vi "SAOMM-SendSET.vi"(0 "PRAMMS-COMM IN":refnum<visa-resource-name>="Hp\u0000\u0002", 1 "Active Refnum":refnum<vi>, 2 "PrAMS-ACK":refnum<vi>, 7 "Signature":u32=1886544237, 11 "Error IN":errorcluster, 12 "MessageType":cluster{string[], u32[]}={["emtError", "emtAreYouThere", "emtAcknowledgment", "emtGetClientType", "emtClientType", "emtGetImageExposureTime", "emtSetImageExposureTime", "emtImageExposureTime", "emtGetOptimalExposureTime", "emtSetOptimalExposureTime", "emtOptimalExposureTime", "emtGetImageEMGain", "emtSetImageEMGain", "emtImageEMGain", "emtGetFPGACtrl", "emtSetFPGACtrl", "emtFPGACtrl", "emtGetImageWidth", "emtSetImageWidth", "emtImageWidth", "emtGetImageHeight", "emtSetImageHeight", "emtImageHeight", "emtGetImageBinning", "emtSetImageBinning", "emtImageBinning", "emtGetImageDisplayFrameRate", "emtSetImageDisplayFrameRate", "emtImageDisplayFrameRate", "emtGetROIWidth", "emtSetROIWidth", "emtROIWidth", "emtGetROIHeight", "emtSetROIHeight", "emtROIHeight", "emtGetROIXOffset", "emtSetROIXOffset", "emtROIXOffset", "emtGetROIYOffset", "emtSetROIYOffset", "emtROIYOffset", "emtStartAcquisition", "mtStopAcquisition", "emtAcquisitionStarted", "emtAcquisitionStopped", "emtGetFalconImage", "emtFalconImage"], [1, 2, 3, 4, 5, 1001, 1101, 1201, 1002, 1102, 1202, 1003, 1103, 1203, 1004, 1104, 1204, 1005, 1105, 1205, 1006, 1106, 1206, 1007, 1107, 1207, 1008, 1108, 1208, 1009, 1109, 1209, 1010, 1110, 1210, 1011, 1111, 1211, 1012, 1112, 1212, 1130, 1131, 1150, 1151, 1070, 1270]}, 13 "Active SET":string="emtSetImageBinning", 14 "Value (little endianed byte array)":u8[](array[numeric])=[2, 0]) -> (4 "PRAMMS-COMM OUT":refnum<visa-resource-name>, 8 "Error":bool, 10 "WaitACKTime":u32=28, 15 "Error OUT":errorcluster)   [LabVIEW 2019]
panel:
  out "CloseTime":u32=5
  out "WriteTime":u32
  out "SortTime":u32
  out "Wait4Flag":u32=27
  out "TotalExec":u32=60
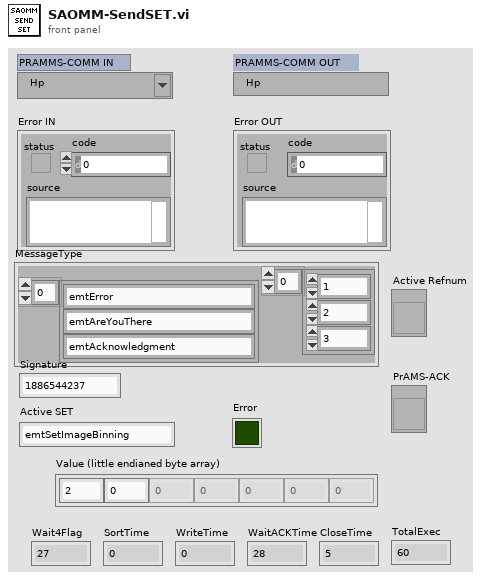
[diagram p1: front panel]
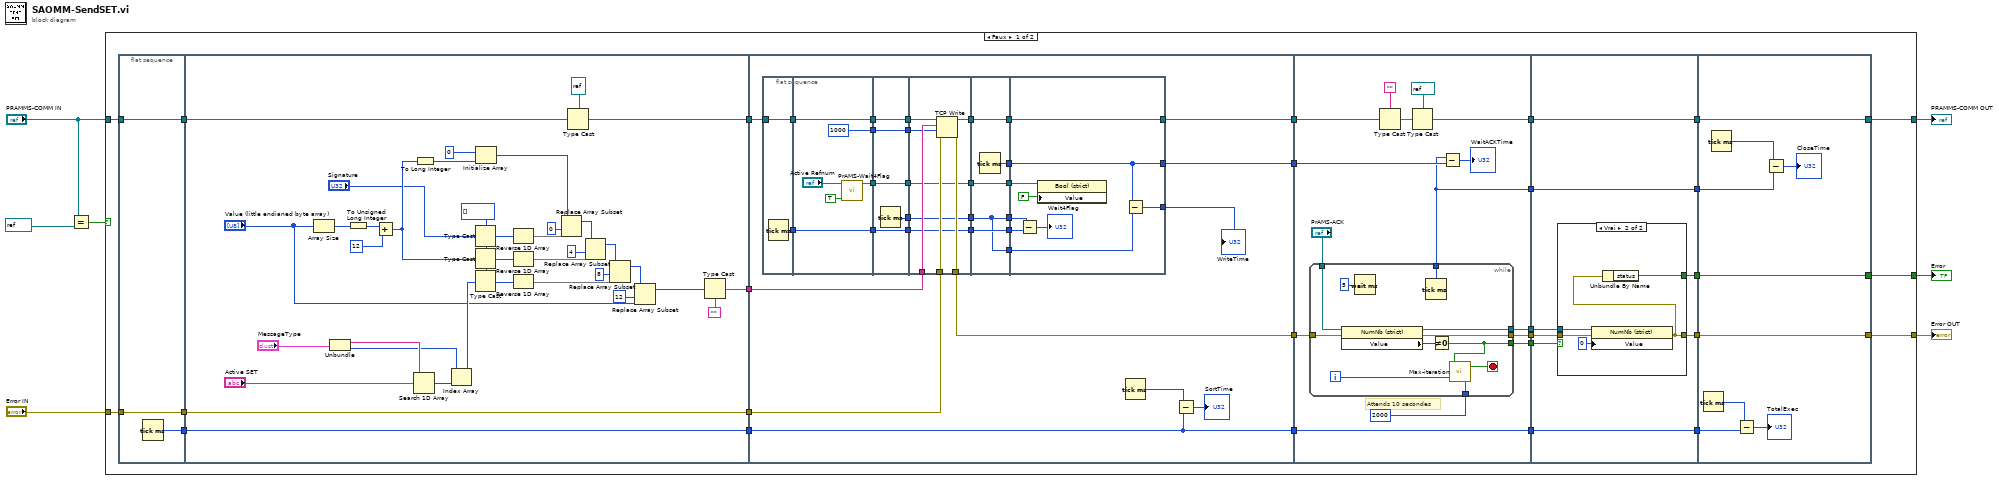
[diagram p0: block diagram]
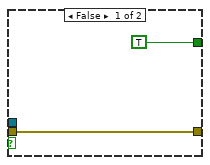
[diagram p2: hidden frame]
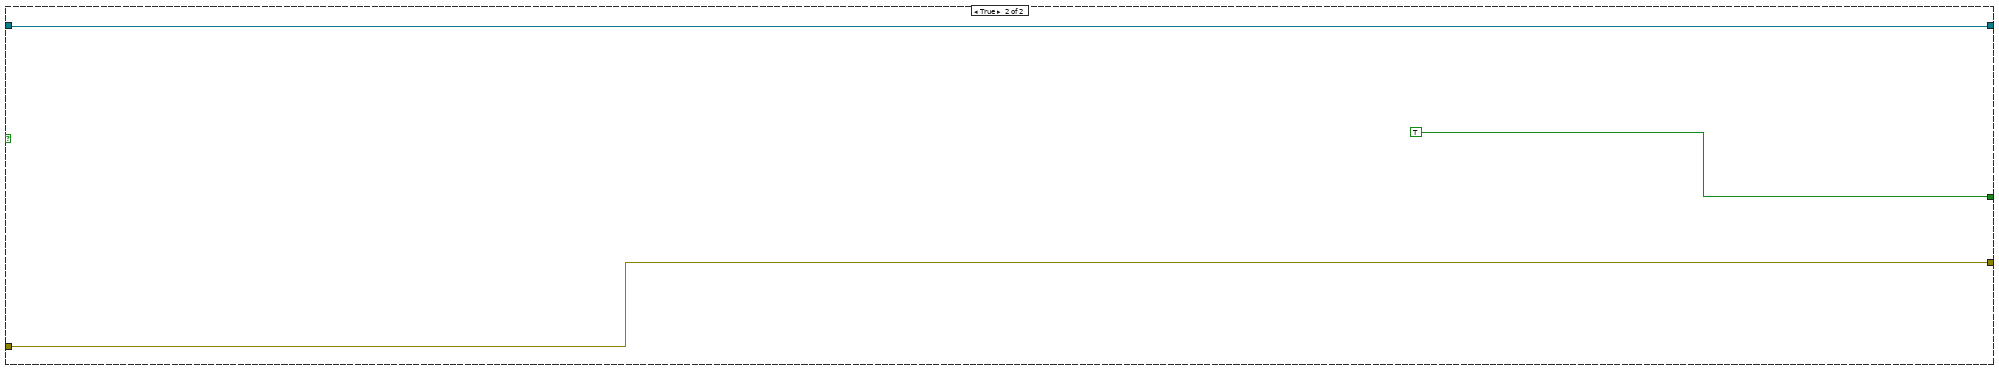
[diagram p3: hidden frame]
diagram:
  n1 = Equal?(x="PRAMMS-COMM IN", y=refnum<visa-resource-name> "-1") -> (x = y?=w4:bool)
  n2 = case shown="Faux" w4 {
    tunnel: "Error IN" -> [w30 w193]
    tunnel: "PRAMMS-COMM IN" -> [w29 w194]
    tunnel: [w28 w193] -> w6
    tunnel: [w14 w194] -> w5
    tunnel: [w27 TRUE] -> w1
    frame False {
      n3 = flat-sequence {
        tunnel: w29 -> [w36]
        tunnel: w30 -> [w37]
        tunnel: [w37] -> w26
        tunnel: [w36] -> w25
        tunnel: [w35] -> w19
        tunnel: w26 -> [w41]
        tunnel: w25 -> [w45]
        tunnel: [w44] -> w16
        tunnel: w19 -> [w44]
        tunnel: [w43] -> w12
        tunnel: [w42] -> w11
        tunnel: [w41] -> w10
        tunnel: [w99] -> w18
        tunnel: [w98] -> w17
        tunnel: w16 -> [w96]
        tunnel: [w96] -> w15
        tunnel: [w103] -> w13
        tunnel: w12 -> [w102]
        tunnel: w11 -> [w101]
        tunnel: w10 -> [w100]
        tunnel: [w156] -> w34
        tunnel: [w155] -> w33
        tunnel: w18 -> [w154]
        tunnel: [w153] -> w32
        tunnel: [w146] -> w31
        tunnel: w17 -> [w151]
        tunnel: [w150] -> w20
        tunnel: w15 -> [w150]
        tunnel: w13 -> [w145]
        tunnel: [w144] -> w8
        tunnel: w34 -> [w174]
        tunnel: w33 -> [w175]
        tunnel: w32 -> [w173]
        tunnel: w31 -> [w171]
        tunnel: [w172] -> w24
        tunnel: [w171] -> w23
        tunnel: [w170] -> w22
        tunnel: [w169] -> w21
        tunnel: w20 -> [w169]
        tunnel: [w168] -> w9
        tunnel: w8 -> [w168]
        tunnel: [w189] -> w27
        tunnel: [w190] -> w14
        tunnel: [w191] -> w28
        tunnel: w24 -> [w191]
        tunnel: w23 -> [w190]
        tunnel: w22 -> [w189]
        tunnel: w21 -> [w188]
        tunnel: w9 -> [w184]
        frame #0 {
          n4 = Tick Count (ms)() -> (millisecond timer value=w35:u32)
        }
        frame #1 {
          w53 = u8[] []
          n5 = Array Size(array="Value (little endianed byte array)") -> (size(s)=w52:i32)
          n6 = Unbundle("MessageType") -> (w39:string[], w38:u32[])
          n7 = To Unsigned Long Integer(number=w52) -> (unsigned 32bit integer=w73:u32)
          n8 = Add(x=w73, y=u32 12 ("x")) -> (x+y=w58:u32)
          n9 = Search 1D Array(1D array=w39, element="Active SET") -> (index of element=w51:i32)  [unwired: 1 in]
          n10 = To Long Integer(number=w58) -> (32bit integer=w59:i32)
          n11 = Index Array(array=w38, index=w51) -> (element=w49:u32)
          n12 = Type Cast(type=w53, x="Signature") -> (*(type *) &x=w56:u8[])
          n13 = Type Cast(type=w53, x=w58) -> (*(type *) &x=w54:u8[])
          n14 = Type Cast(type=w53, x=w49) -> (*(type *) &x=w55:u8[])
          n15 = Initialize Array(u8 0, w59) -> (w67:u8[])
          n16 = Reverse 1D Array(array=w56) -> (reversed array=w70:u8[])
          n17 = Reverse 1D Array(array=w54) -> (reversed array=w71:u8[])
          n18 = Reverse 1D Array(array=w55) -> (reversed array=w72:u8[])
          n19 = Replace Array Subset(array=w67, new element=w70, index=0) -> (w60:u8[])
          n20 = Type Cast(type=refnum<k5> refnum ("connection ID"), x=w45) -> (*(type *) &x=w43:refnum<k5>)
          n21 = Replace Array Subset(array=w60, new element=w71, index=4) -> (w61:u8[])
          n22 = Replace Array Subset(array=w61, new element=w72, index=8) -> (w62:u8[])
          n23 = Replace Array Subset(array=w62, new element="Value (little endianed byte array)", index=12) -> (w68:u8[])
          n24 = Type Cast(type="", x=w68) -> (*(type *) &x=w42:string)
        }
        frame #2 {
          n25 = flat-sequence {
            tunnel: w102 -> [w107]
            tunnel: [w107] -> w105
            tunnel: [w106] -> w104
            tunnel: [w113] -> w94
            tunnel: [w110] -> w92
            tunnel: w105 -> [w113]
            tunnel: [w109] -> w90
            tunnel: w104 -> [w109]
            tunnel: [1000 ("timeout ms (25000)")] -> w88
            tunnel: w94 -> [w118]
            tunnel: [w118] -> w93
            tunnel: w92 -> [w117]
            tunnel: [w117] -> w91
            tunnel: w90 -> [w116]
            tunnel: [w116] -> w89
            tunnel: w88 -> [w115]
            tunnel: [w115] -> w87
            tunnel: [w114] -> w86
            tunnel: w101 -> [w127]
            tunnel: w100 -> [w124]
            tunnel: [w123] -> w99
            tunnel: [w126] -> w85
            tunnel: w93 -> [w125]
            tunnel: [w122] -> w83
            tunnel: w91 -> [w122]
            tunnel: [w119] -> w81
            tunnel: [w121] -> w79
            tunnel: w89 -> [w121]
            tunnel: w87 -> [w120]
            tunnel: w86 -> [w119]
            tunnel: w85 -> [w132]
            tunnel: [w132] -> w84
            tunnel: w83 -> [w131]
            tunnel: [w131] -> w82
            tunnel: w81 -> [w128]
            tunnel: [w128] -> w80
            tunnel: w79 -> [w130]
            tunnel: [w130] -> w78
            tunnel: [w128] -> w77
            tunnel: [w129] -> w76
            tunnel: [w141] -> w103
            tunnel: w84 -> [w141]
            tunnel: w82 -> [w140]
            tunnel: [w134] -> w98
            tunnel: w80 -> [w137]
            tunnel: w78 -> [w138]
            tunnel: w77 -> [w135]
            tunnel: w76 -> [w134]
            tunnel: [w133] -> w75
            frame #0 {
              n26 = Tick Count (ms)() -> (millisecond timer value=w106:u32)
            }
            frame #1 {
              n27 = call "PrAMS-Wait4Flag.vi"("Raise Flag ?"=TRUE, "Ctl Refnum IN"="Active Refnum") -> ("Ctl Refnum OUT"=w110:refnum<vi>)  [unwired: 8 in, 1 out]
            }
            frame #2 {
              n28 = Tick Count (ms)() -> (millisecond timer value=w114:u32)
            }
            frame #3 {
              n29 = TCP Write(connection ID=w125, data in=w127, error in (no error)=w124, 9:w120) -> (connection ID out=w126:refnum<k5>, error out=w123:errorcluster)  [unwired: 1 out]
            }
            frame #4 {
              n30 = Tick Count (ms)() -> (millisecond timer value=w129:u32)
            }
            frame #5 {
              n31 = Subtract(x=w137, y=w138) -> (x-y=→"Wait4Flag":u32)
              n32 = property class="Bool (strict)"(reference=w140, "Value"=FALSE ("Raise Flag ?")) -> ()  [unwired: 1 in, 2 out]
              n33 = Subtract(x=w134, y=w135) -> (x-y=w133:u32)
            }
          }
          n34 = Tick Count (ms)() -> (millisecond timer value=w97:u32)
          n35 = Subtract(x=w97, y=w96) -> (x-y=→"SortTime":u32)
          "WriteTime" <- w75
        }
        frame #3 {
          # "Attends 10 secondes"
          n36 = while {
            tunnel: [w159] -> w156
            tunnel: [w161] -> w155
            tunnel: w154 -> [w162]
            tunnel: [w160] -> w153
            tunnel: [w164] -> w144
            tunnel: "PrAMS-ACK" -> [w163]
            tunnel: 2000 ("i max") -> [w158]
            i -> [w167]
            stop <- w166 stop-if-true
            n37 = property class="NumNb (strict)"(reference=w163, error in=w162) -> (reference out=w161:refnum<vi>, error out=w160:errorcluster, "Value"=w157:i32)
            n38 = Wait (ms)(milliseconds to wait=u32 5) -> ()  [unwired: 1 out]
            n39 = Tick Count (ms)() -> (millisecond timer value=w164:u32)
            n40 = Not Equal To 0?(x=w157) -> (x != 0?=w159:bool)
            n41 = call "Max-iteration.vi"("i max"=w158, "i act"=w167, "Valeur entrante"=w159) -> ("break ?"=w166:bool)
          }
          n42 = Type Cast(type="", x=w145) -> (*(type *) &x=w147:string)
          n43 = Type Cast(type=refnum<visa-resource-name> refnum ("PRAMMS-COMM IN"), x=w147) -> (*(type *) &x=w146:refnum<visa-resource-name>)
          n44 = Subtract(x=w144, y=w151) -> (x-y=→"WaitACKTime":u32)
        }
        frame #4 {
          n45 = case shown="Vrai" w174 {
            tunnel: w175 -> [_ w182]
            tunnel: w173 -> [w176 w181]
            tunnel: [w176 w180] -> w172
            tunnel: [TRUE w179] -> w170
            frame False {
            }
            frame True {
              n46 = property class="NumNb (strict)"(reference=w182, error in=w181, "Value"=0) -> (error out=w180:errorcluster)  [unwired: 1 out]
              n47 = Unbundle By Name(w180) -> ("status"=w179:bool)
            }
          }
        }
        frame #5 {
          n48 = Tick Count (ms)() -> (millisecond timer value=w187:u32)
          n49 = Tick Count (ms)() -> (millisecond timer value=w183:u32)
          n50 = Subtract(x=w187, y=w188) -> (x-y=→"TotalExec":u32)
          n51 = Subtract(x=w183, y=w184) -> (x-y=→"CloseTime":u32)
        }
      }
    }
    frame True {
    }
  }
  "Error OUT" <- w6
  "Error" <- w1
  "PRAMMS-COMM OUT" <- w5
